vi "Conveyer Belt Get.vi"(1 "Vertical Belt":dbl, 2 "Horizontal Belt":dbl) -> ()   [LabVIEW 2012]
uses:
  Conveyer Belt Global Data.vi
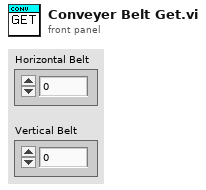
[diagram p1: front panel]
types:
  T1 = cluster{"Horizontal Belt":dbl, "Vertical Belt":dbl, "MS":bool}
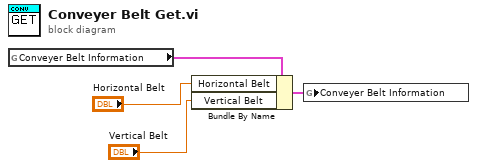
[diagram p0: block diagram]
diagram:
  n1 = global read "Conveyer Belt Global Data.vi" "Conveyer Belt Information"() -> (w3:T1)
  n2 = Bundle By Name(cluster=w3, "Horizontal Belt"="Horizontal Belt", "Vertical Belt"="Vertical Belt") -> (w4:T1)
  n3 = global write "Conveyer Belt Global Data.vi" "Conveyer Belt Information"(w4) -> ()
